vi "Periodic Tasks.vi"(8 "error in (no error)":errorcluster) -> ()   [LabVIEW 2013]
doc: "This VI runs in parallel to other tasks. It can contain as many user-defined periodic loops as you need. These can carry out PID or other sorts of timed response."
uses:
  TankDriveEnum.ctl
  <vilib>/Rock Robotics/SystemInterfaces/Utilities/FPGA_UtilitiesLED Source.ctl
  <vilib>/Rock Robotics/SystemInterfaces/Utilities/FPGA_UtilitiesLED State.ctl
  <vilib>/Rock Robotics/WPI/Solenoid/WPI_SolenoidValue.ctl
  <vilib>/Rock Robotics/WPI/Compressor/WPI_CompressorGetSetRefNum.vi
  Robot Global Data.vi
  <vilib>/Rock Robotics/WPI/Solenoid/WPI_SolenoidSetEnum.vi
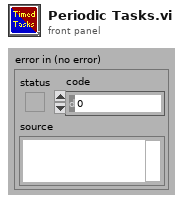
[diagram p1: front panel]
types:
  T1 = typedef "FPGA_UtilitiesLED State.ctl" = enum16{"Off", "On", "Toggle"}
  T2 = typedef "FPGA_UtilitiesLED Source.ctl" = enum16{"User LED", "FPGA LED"}
  T3 = typedef "WPI_EncoderDevRef.ctl" = cluster{"DevStatus":errorcluster, "EncoderIndex":T4, "CounterIndex":T5, "DistancePerCount":dbl, "Decoding Type":T6}
  T4 = typedef "FPGA_EncoderIdx.ctl" = enum8{"Enc 0", "Enc 1", "Enc 2", "Enc 3", "Invalid"}
  T5 = typedef "FPGA_CounterCtrSystemIndex.ctl" = enum8{"Ctr 0", "Ctr 1", "Ctr 2", "Ctr 3", "Ctr 4", "Ctr 5", "Ctr 6", "Ctr 7", "Invalid"}
  T6 = typedef "WPI_EncoderType.ctl" = enum16{"1x", "2x", "4x"}
  T7 = typedef "WPI_CompressorDevRef.ctl" = cluster{"DevStatus":errorcluster, "DigitalInputDevRef":T8, "RelayDevRef":T11}
  T8 = typedef "WPI_DigitalInputDevRef.ctl" = cluster{"DevStatus":errorcluster, "DIO Channel":T9, "Digital Module":T10}
  T9 = typedef "FPGA_DIOChannel.ctl" = enum8{"DIO 1", "DIO 2", "DIO 3", "DIO 4", "DIO 5", "DIO 6", "DIO 7", "DIO 8", "DIO 9", "DIO 10", "DIO 11", "DIO 12", "DIO 13", "DIO 14", "Invalid"}
  T10 = typedef "FPGA_TypedefDigitalModule.ctl" = enum16{"Digital Module 1", "Digital Module 2"}
  T11 = typedef "WPI_RelayDevRef.ctl" = cluster{"DevStatus":errorcluster, "Relay Channel":T12, "Digital Module":T10, "Relay Direction":T13}
  T12 = typedef "FPGA_DIORelayChannel.ctl" = enum8{"Relay 1", "Relay 2", "Relay 3", "Relay 4", "Relay 5", "Relay 6", "Relay 7", "Relay 8", "Invalid"}
  T13 = typedef "WPI_RelayDirection.ctl" = enum16{"Both directions", "Forward only", "Reverse only"}
  T14 = typedef "WPI_SolenoidDevRef.ctl" = cluster{"DevStatus":errorcluster, "Solenoid Module":T15, "Forward Solenoid Channel":T16, "Reverse Solenoid Channel":T16}
  T15 = typedef "FPGA_TypedefSolenoidModule.ctl" = enum16{"Solenoid Module 1", "Solenoid Module 2"}
  T16 = typedef "WPI_SolenoidChannel.ctl" = enum8{"Solenoid 1", "Solenoid 2", "Solenoid 3", "Solenoid 4", "Solenoid 5", "Solenoid 6", "Solenoid 7", "Solenoid 8", "Invalid"}
  T17 = typedef "TankDriveEnum.ctl" = enum16{"Init", "SetValue", "Disable", "Linear Drive"}
  T18 = typedef "WPI_SolenoidValue.ctl" = enum16{"Off", "On", "Forward", "Reverse"}
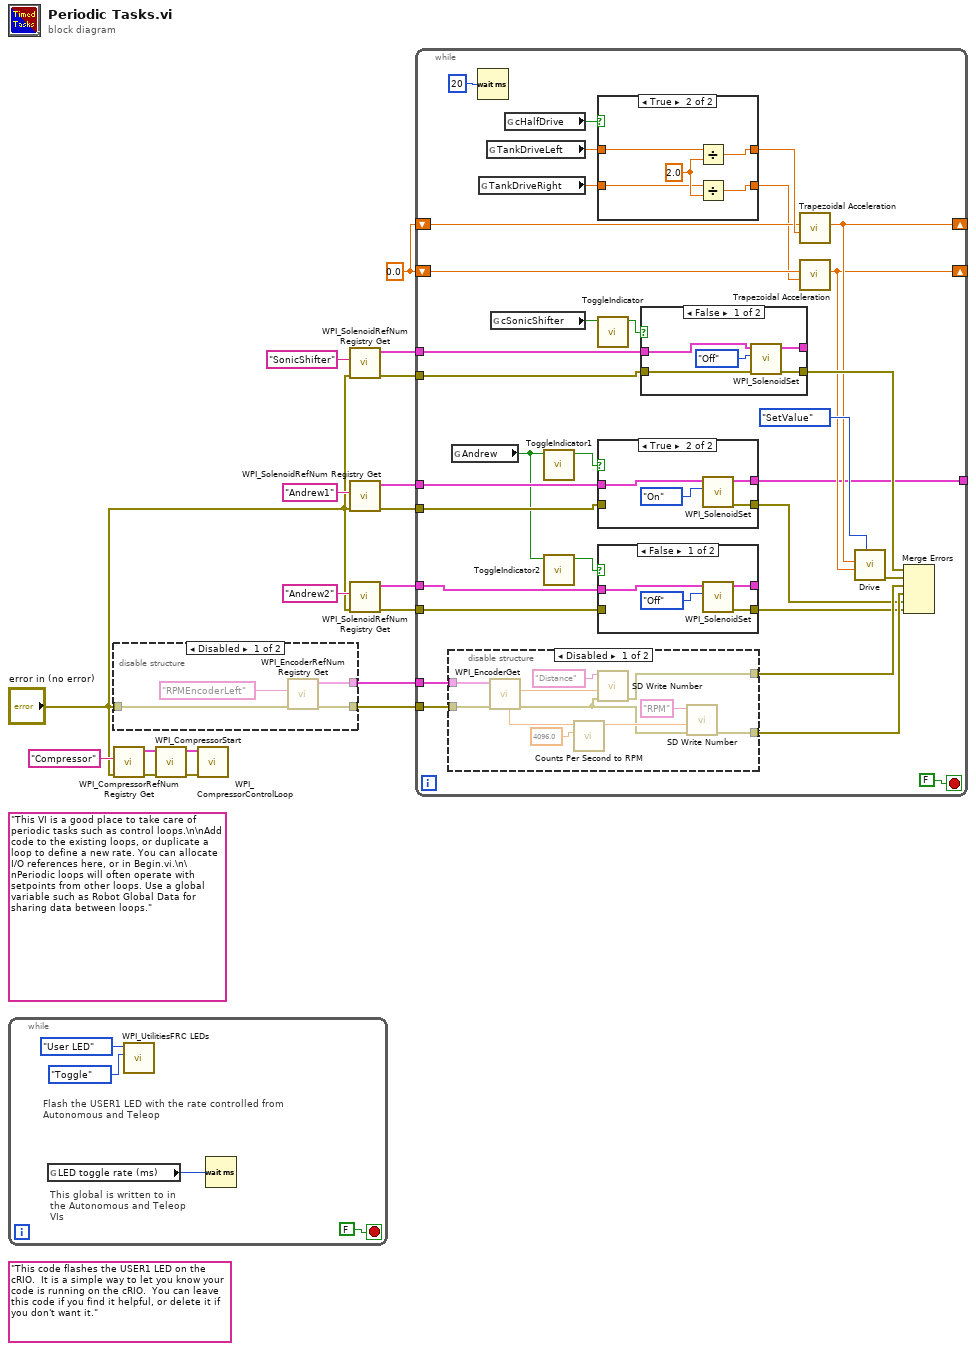
[diagram p0: block diagram]
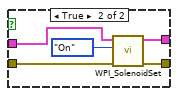
[diagram p3: hidden frame]
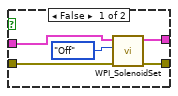
[diagram p4: hidden frame]
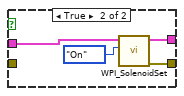
[diagram p7: hidden frame]
diagram:
  w12 = 0.0
  (unwired) "This code flashes the USER1 LED on the cRIO.  It is a simple way to let you know your code is running on the cRIO.  You can leave this code if you find it helpful, or delete it if you don't want it."
  (unwired) "This VI is a good place to take care of periodic tasks such as control loops.\n\nAdd code to the existing loops, or duplicate a loop to define a new rate. You can allocate I/O references here, or in Begin.vi.\n\nPeriodic loops will often operate with setpoints from other loops. Use a global variable such as Robot Global Data for sharing data between loops."
  n1 = while {
    stop <- FALSE stop-if-true
    # "This global is written to in the Autonomous and Teleop VIs"
    # "Flash the USER1 LED with the rate controlled from Autonomous and Teleop"
    n2 = global read "Robot Global Data.vi" "LED toggle rate (ms)"() -> (w19:u32)
    n3 = call <vilib>:"WPI_UtilitiesFRC LEDs.vi"("State"=FPGA_UtilitiesLED_State."Toggle", "LED Type"=FPGA_UtilitiesLED_Source."User LED") -> ()  [unwired: 1 in, 9 out]
    n4 = Wait (ms)(milliseconds to wait=w19) -> ()  [unwired: 1 out]
  }
  n5 = disable-structure shown="Disabled" {
    disable-tunnel: [w25 _] -> w10
    disable-tunnel: [w24 _] -> w9
    disable-tunnel: "error in (no error)" -> [w23 _]
    frame Disabled {
      n6 = call <vilib>:"WPI_EncoderRefNum Registry Get.vi"("error in (no error)"=w23, "refnum name"="RPMEncoderLeft") -> ("error out"=w24:errorcluster, "EncoderDevRef"=w25:T3)  [unwired: 8 in]
    }
    frame Enabled {
    }
  }
  n7 = call <vilib>:"WPI_CompressorRefNum Registry Get.vi"("error in (no error)"="error in (no error)", "refnum name"="Compressor") -> ("error out"=w15:errorcluster, "CompressorDevRef"=w18:T7)  [unwired: 8 in]
  n8 = call <vilib>:"WPI_CompressorStart.vi"("error in (no error)"=w15, "CompressorDevRef"=w18) -> ("error out"=w11:errorcluster, "CompressorDevRef"=w17:T7)  [unwired: 8 in]
  n9 = call <vilib>:"WPI_CompressorControlLoop.vi"("error in (no error)"=w11, "CompressorDevRef"=w17) -> ()  [unwired: 10 in]
  n10 = call <vilib>:"WPI_SolenoidRefNum Registry Get.vi"("error in (no error)"="error in (no error)", "refnum name"="SonicShifter") -> ("error out"=w8:errorcluster, "SolenoidDevRef"=w13:T14)  [unwired: 8 in]
  n11 = call <vilib>:"WPI_SolenoidRefNum Registry Get.vi"("error in (no error)"="error in (no error)", "refnum name"="Andrew1") -> ("error out"=w2:errorcluster, "SolenoidDevRef"=w5:T14)  [unwired: 8 in]
  n12 = call <vilib>:"WPI_SolenoidRefNum Registry Get.vi"("error in (no error)"="error in (no error)", "refnum name"="Andrew2") -> ("error out"=w1:errorcluster, "SolenoidDevRef"=w4:T14)  [unwired: 8 in]
  n13 = while {
    tunnel: w13 -> [w55]
    shift-right: [w43] -> _
    shift-left: w12 -> [w46]
    shift-right: [w42] -> _
    shift-left: w12 -> [w45]
    tunnel: w10 -> [w41]
    tunnel: w9 -> [w40]
    tunnel: w8 -> [w39]
    tunnel: w5 -> [w34]
    tunnel: w4 -> [w33]
    tunnel: w2 -> [w32]
    tunnel: w1 -> [w31]
    tunnel: [w28] -> _
    stop <- FALSE stop-if-true
    n14 = disable-structure shown="Disabled" {
      disable-tunnel: w41 -> [w87 _]
      disable-tunnel: w40 -> [w86 _]
      disable-tunnel: [w78 _] -> w38
      disable-tunnel: [w77 _] -> w37
      frame Disabled {
        n15 = call <vilib>:"WPI_EncoderGet.vi"("error in (no error)"=w86, "EncoderDevRef"=w87) -> ("error out"=w80:errorcluster, "Distance"=w81:dbl, "Rate"=w85:dbl)  [unwired: 4 in, 3 out]
        n16 = call "Counts Per Second to RPM.vi"("Counts/Rev"=4096.0, "Counts/Second"=w85) -> ("RPM"=w83:dbl)  [unwired: 9 in]
        n17 = call <vilib>:"SD Write Number.vi"("error in"=w80, "Numeric"=w81, "Name"="Distance") -> ("error out"=w78:errorcluster)  [unwired: 7 in, 1 out]
        n18 = call <vilib>:"SD Write Number.vi"("error in"=w80, "Numeric"=w83, "Name"="RPM") -> ("error out"=w77:errorcluster)  [unwired: 7 in, 1 out]
      }
      frame Enabled {
      }
    }
    n19 = global read "Robot Global Data.vi" "Andrew"() -> (w27:bool)
    n20 = Wait (ms)(milliseconds to wait=u32 20) -> ()  [unwired: 1 out]
    n21 = global read "Robot Global Data.vi" "TankDriveRight"() -> (w52:dbl)
    n22 = global read "Robot Global Data.vi" "TankDriveLeft"() -> (w51:dbl)
    n23 = global read "Robot Global Data.vi" "cSonicShifter"() -> (w57:bool)
    n24 = global read "Robot Global Data.vi" "cHalfDrive"() -> (w50:bool)
    n25 = call "ToggleIndicator1.vi"("cSonicShifter"=w27) -> ("Actuate?"=w36:bool)  [unwired: 10 in]
    n26 = call "ToggleIndicator2.vi"("cSonicShifter"=w27) -> ("Actuate?"=w35:bool)  [unwired: 10 in]
    n27 = case shown="True" w50 {
      tunnel: w52 -> [w88 w93]
      tunnel: w51 -> [w89 w92]
      tunnel: [w89 w91] -> w47
      tunnel: [w88 w90] -> w44
      frame False {
      }
      frame True {
        w94 = 2.0
        n28 = Divide(x=w92, y=w94) -> (x/y=w91:dbl)
        n29 = Divide(x=w93, y=w94) -> (x/y=w90:dbl)
      }
    }
    n30 = call "ToggleIndicator.vi"("cSonicShifter"=w57) -> ("Actuate?"=w56:bool)  [unwired: 10 in]
    n31 = case shown="True" w36 {
      tunnel: [w71 w75] -> w28
      tunnel: [w70 w74] -> w30
      tunnel: w34 -> [w69 w73]
      tunnel: w32 -> [w68 _]
      frame False {
        n32 = call-poly <vilib>:"WPI_SolenoidSet.vi"("error in (no error)"=w68, "Value"=WPI_SolenoidValue."Off", "SolenoidDevRef"=w69) -> ("error out"=w70:errorcluster, "SolenoidDevRef"=w71:T14)  [unwired: 7 in]
      }
      frame True {
        n33 = call-poly <vilib>:"WPI_SolenoidSet.vi"("Value"=WPI_SolenoidValue."On", "SolenoidDevRef"=w73) -> ("error out"=w74:errorcluster, "SolenoidDevRef"=w75:T14)  [unwired: 8 in]
      }
    }
    n34 = case shown="False" w35 {
      tunnel: [w61 w66] -> _
      tunnel: [w60 w65] -> w29
      tunnel: w33 -> [w59 w64]
      tunnel: w31 -> [_ w63]
      frame False {
        n35 = call-poly <vilib>:"WPI_SolenoidSet.vi"("Value"=WPI_SolenoidValue."Off", "SolenoidDevRef"=w59) -> ("error out"=w60:errorcluster, "SolenoidDevRef"=w61:T14)  [unwired: 8 in]
      }
      frame True {
        n36 = call-poly <vilib>:"WPI_SolenoidSet.vi"("error in (no error)"=w63, "Value"=WPI_SolenoidValue."On", "SolenoidDevRef"=w64) -> ("error out"=w65:errorcluster, "SolenoidDevRef"=w66:T14)  [unwired: 7 in]
      }
    }
    n37 = case shown="False" w56 {
      tunnel: [w98 w102] -> _
      tunnel: w55 -> [w97 w101]
      tunnel: [w96 w100] -> w49
      tunnel: w39 -> [w95 _]
      frame False {
        n38 = call-poly <vilib>:"WPI_SolenoidSet.vi"("error in (no error)"=w95, "Value"=WPI_SolenoidValue."Off", "SolenoidDevRef"=w97) -> ("error out"=w96:errorcluster, "SolenoidDevRef"=w98:T14)  [unwired: 7 in]
      }
      frame True {
        n39 = call-poly <vilib>:"WPI_SolenoidSet.vi"("Value"=WPI_SolenoidValue."On", "SolenoidDevRef"=w101) -> ("error out"=w100:errorcluster, "SolenoidDevRef"=w102:T14)  [unwired: 8 in]
      }
    }
    n40 = call "Trapezoidal Acceleration.vi"("Desired"=w47, "Actual"=w46) -> ("New Actual"=w43:dbl)  [unwired: 9 in]
    n41 = call "Trapezoidal Acceleration.vi"("Desired"=w44, "Actual"=w45) -> ("New Actual"=w42:dbl)  [unwired: 9 in]
    n42 = call "Drive.vi"("Enum"=TankDriveEnum."SetValue", "Right"=w42, "Left"=w43) -> ("error out"=w48:errorcluster)  [unwired: 8 in]
    n43 = Merge Errors(w49, w48, w38, w37, w30, w29) -> ()  [unwired: 1 out]
  }
